vi "Set Plugin Configurations.vi"(10 "Plugin Configurations":refnum<class "Plugin Configuration.lvclass">[](array[class]), 11 "Framework Configuration in":refnum<class "Framework Configuration.lvclass">) -> (3 "Framework Configuration out":refnum<class "Framework Configuration.lvclass">)   [LabVIEW 2017, in "DSF Core.lvlib" / "Framework Configuration.lvclass"]
uses:
  Framework Configuration.lvclass
  Plugin/Plugin Configuration.lvclass
  Framework Configuration.lvclass/Framework Configuration.ctl
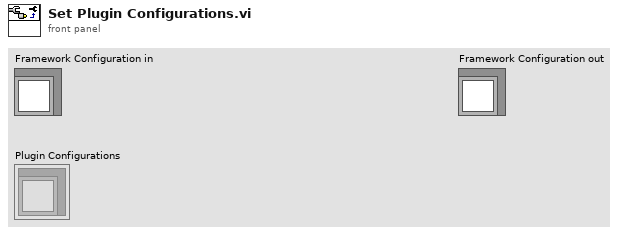
[diagram p1: front panel]
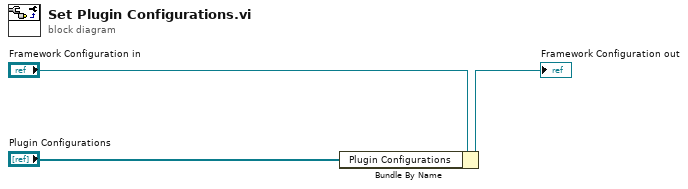
[diagram p0: block diagram]
diagram:
  n1 = Bundle By Name(cluster="Framework Configuration in", "Plugin Configurations"="Plugin Configurations") -> (→"Framework Configuration out":refnum<class "Framework Configuration.lvclass">)
